vi "sm u32 read and increment.vi"(8 "Identifier":string, 11 "Shared memory cluster input":T1) -> (2 "Value out":u32, 3 "Shared memory cluster output":T1)   [LabVIEW 2020, in "linuxSharedMemory.lvlib"]
uses:
  linuxSharedMemory.lvlib
  controls/sm_cluster.ctl
  <vilib>/NI/NI Linux RT IPC/Shared Memory/Pointer Operations/Read Scalar U32.vi
  <vilib>/NI/NI Linux RT IPC/Shared Memory/Pointer Operations/In Place Read Pointer.vi
  <vilib>/NI/NI Linux RT IPC/Shared Memory/Pointer Operations/In Place Read Scalar U32.vi
  <vilib>/NI/NI Linux RT IPC/Shared Memory/Linux RT IPC.Shared Memory.lvlib
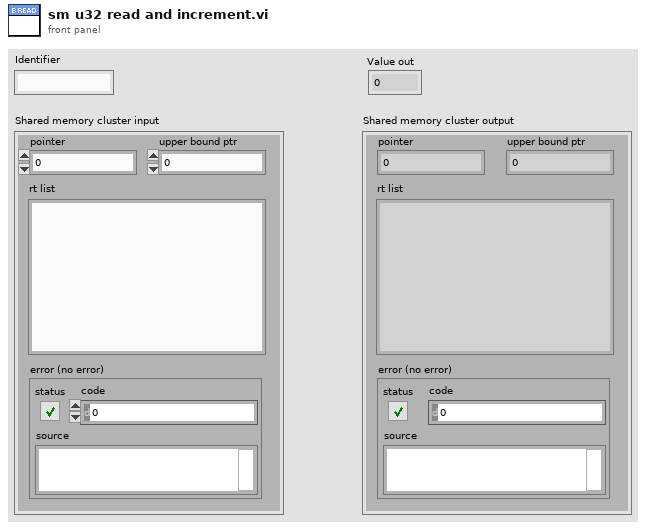
[diagram p1: front panel]
types:
  T1 = typedef "linuxSharedMemory.lvlib/sm_cluster.ctl" = cluster{"rt list":string, "error (no error)":errorcluster, "pointer":u64, "upper bound ptr":u64}
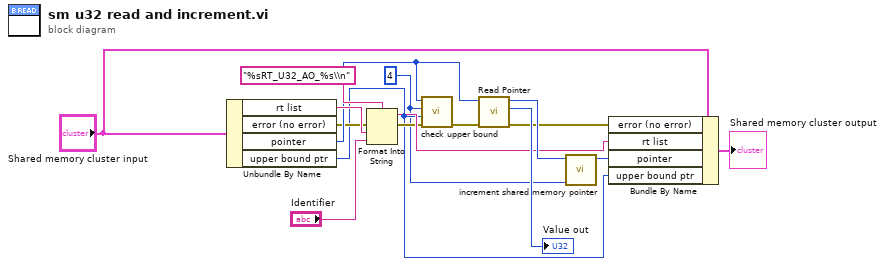
[diagram p0: block diagram]
diagram:
  w1 = 4
  n1 = Unbundle By Name("Shared memory cluster input") -> ("rt list"=w12:string, "error (no error)"=w7:errorcluster, "pointer"=w11:u64, "upper bound ptr"=w4:u64)
  n2 = Format Into String(format string="%sRT_U32_AO_%s\\n", error in=w7, w12, "Identifier") -> (resulting string=w8:string, error out=w6:errorcluster)  [unwired: 1 in]
  n3 = call "check upper bound.vi"("error in (no error)"=w6, "ptr upper bound (inclusive)"=w4, "size"=w1, "ptr in"=w11) -> ("error out"=w10:errorcluster)  [unwired: 7 in]
  n4 = call-poly <vilib>:"Read Pointer.vi"("error in (no error)"=w10, "pointer in"=w11) -> ("error out"=w9:errorcluster, "value out"=→"Value out":u32, "pointer out"=w16:u64)  [unwired: 7 in]
  n5 = call "increment shared memory pointer.vi"("Increment value"=w1, "Shared Memory PTR in"=w16) -> ("Shared Memory PTR out"=w5:u64)  [unwired: 9 in]
  n6 = Bundle By Name(cluster="Shared memory cluster input", "error (no error)"=w9, "rt list"=w8, "pointer"=w5, "upper bound ptr"=w4) -> (→"Shared memory cluster output":T1)
